vi "PicoScope5000aSettings.vi"(0 "error in":errorcluster, 1 "Channel A Settings":T2={"Enabled"=FALSE, "Coupling"=1, "Range"=6, "Analogue Offset"=0.0, "Bandwidth Limit"=0} {"Bandwidth Limit" items=["Full", "20MHz"]; "Range" items=["10 mV", "20 mV", "50 mV", "100 mV", "200 mV", "500 mV", "1 V", "2 V", "5 V", "10 V", "20 V"]; "Coupling" items=["AC", "DC"]}, 2 "Port 0 Settings":cluster{"Enabled":bool, "Logic Level":i16}={"Enabled"=FALSE, "Logic Level"=9830} {"Logic Level" items=["1.5V TTL"=9830, "2.5V CMOS"=16383]}, 3 "Channel B Settings":T2={"Enabled"=FALSE, "Coupling"=1, "Range"=6, "Analogue Offset"=0.0, "Bandwidth Limit"=0} {"Bandwidth Limit" items=["Full", "20MHz"]; "Range" items=["10 mV", "20 mV", "50 mV", "100 mV", "200 mV", "500 mV", "1 V", "2 V", "5 V", "10 V", "20 V"]; "Coupling" items=["AC", "DC"]}, 5 "handle in":i16, 9 "Device Info":T1, 11 "Trigger Settings":T3={"Trigger Enabled"=FALSE, "Trigger Source"=enum."Channel A", "Trigger Threshold (volts)"=0.0, "Trigger Direction"=2, "Trigger Delay (samples)"=0, "Auto Trigger Time (ms)"=1000} {"Trigger Direction" items=["Rising"=2, "Falling"=3]}, 12 "Channel C Settings":T2={"Enabled"=FALSE, "Coupling"=1, "Range"=6, "Analogue Offset"=0.0, "Bandwidth Limit"=0} {"Bandwidth Limit" items=["Full", "20MHz"]; "Range" items=["10 mV", "20 mV", "50 mV", "100 mV", "200 mV", "500 mV", "1 V", "2 V", "5 V", "10 V", "20 V"]; "Coupling" items=["AC", "DC"]}, 13 "Port 1 Settings":cluster{"Enabled":bool, "Logic Level":i16}={"Enabled"=FALSE, "Logic Level"=9830} {"Logic Level" items=["1.5V TTL"=9830, "2.5V CMOS"=16383]}, 14 "Channel D Settings":T2={"Enabled"=FALSE, "Coupling"=1, "Range"=6, "Analogue Offset"=0.0, "Bandwidth Limit"=0} {"Bandwidth Limit" items=["Full", "20MHz"]; "Range" items=["10 mV", "20 mV", "50 mV", "100 mV", "200 mV", "500 mV", "1 V", "2 V", "5 V", "10 V", "20 V"]; "Coupling" items=["AC", "DC"]}, 15 "Max ADC value":i16) -> (4 "error out":errorcluster, 6 "handle out":i16, 8 "enabled array":i16[](array[numeric]))   [LabVIEW 2020]
doc: "This VI is used to set up the oscilloscope. The inputs are clusters for setting channel and simple trigger settings. Advanced triggers can be set up using PicoScope3000aAdvancedTriggerSettings.vi"
uses:
  ps5000a.dll
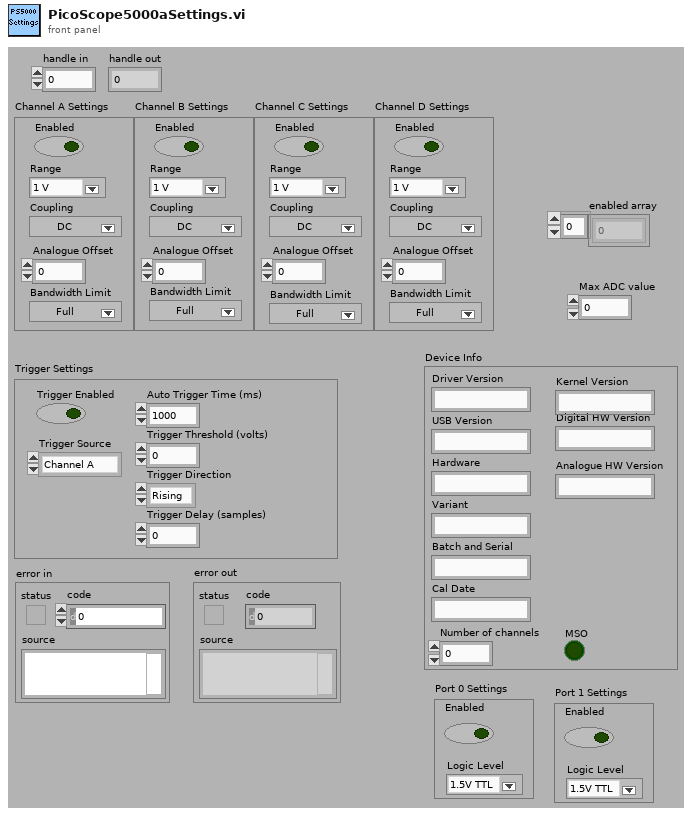
[diagram p1: front panel]
types:
  T1 = cluster{"Driver Version":string, "USB Version":string, "Hardware":string, "Variant":string, "Batch and Serial":string, "Cal Date":string, "Kernel Version":string, "Digital HW Version":string, "Analogue HW Version":string, "MSO":bool, "Number of channels":i16}
  T2 = cluster{"Enabled":bool, "Coupling":i16, "Range":u16, "Analogue Offset":sgl, "Bandwidth Limit":u32}
  T3 = cluster{"Trigger Enabled":bool, "Trigger Source":enum16{"Channel A", "Channel B", "Channel C", "Channel D", "Ext."}, "Trigger Threshold (volts)":dbl, "Trigger Direction":u16, "Trigger Delay (samples)":u32, "Auto Trigger Time (ms)":i16}
  T4 = enum16{"Channel A", "Channel B", "Channel C", "Channel D", "Ext."}
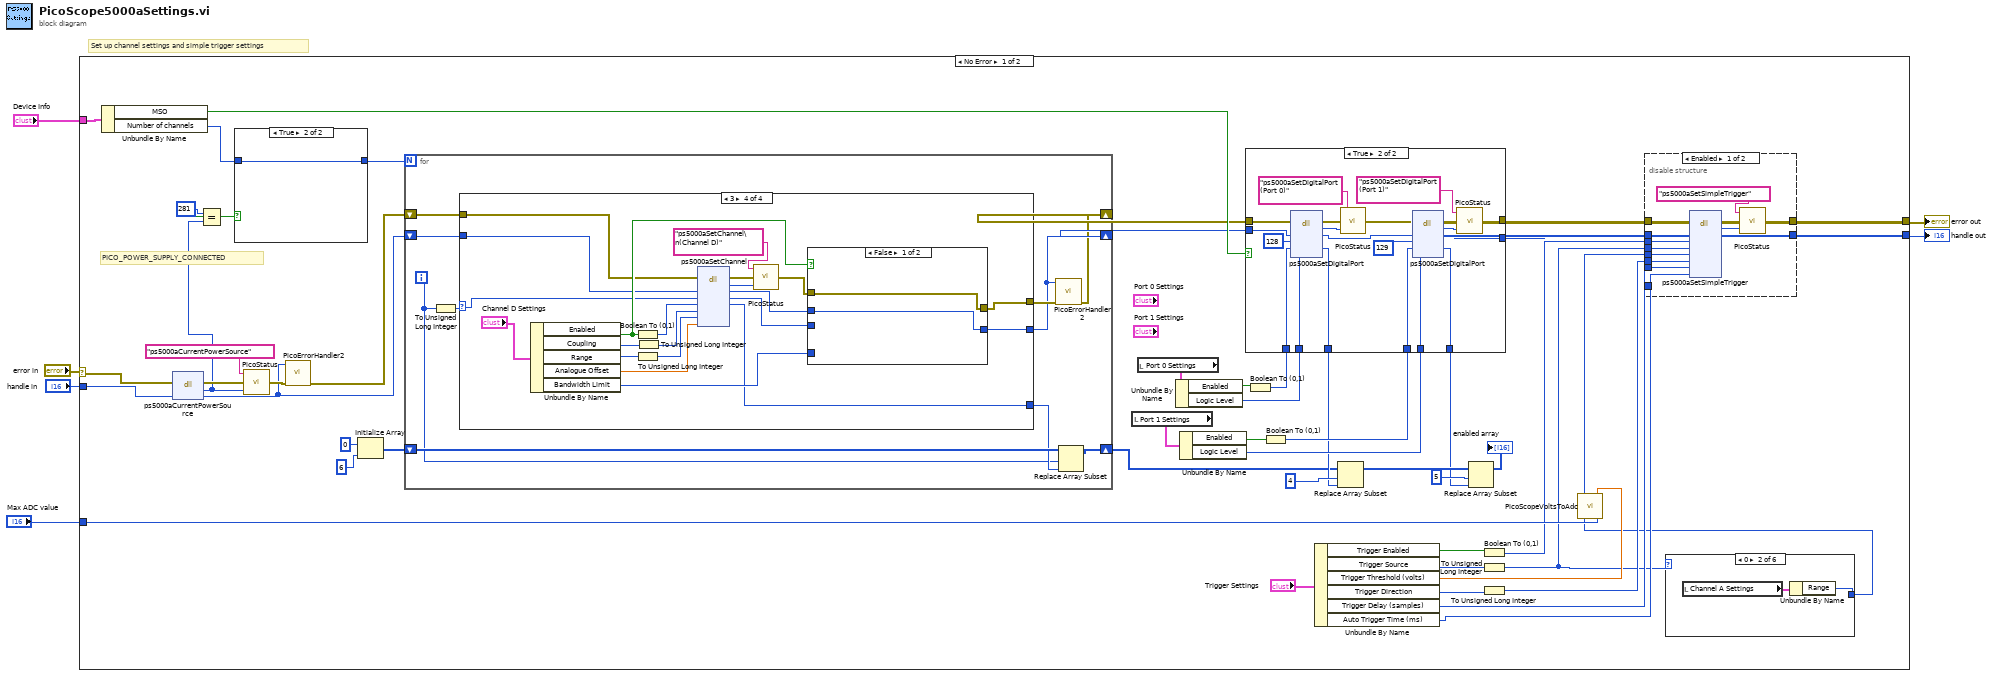
[diagram p0: block diagram]
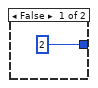
[diagram p3: hidden frame]
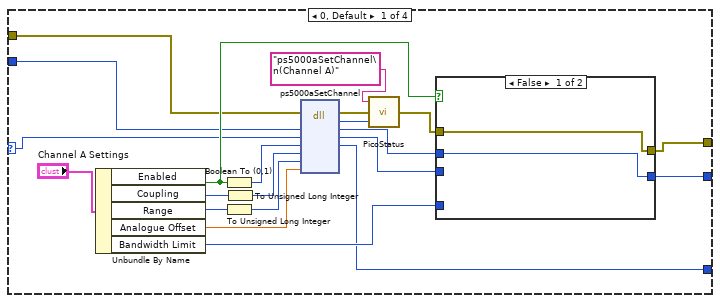
[diagram p4: hidden frame]
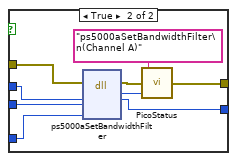
[diagram p5: hidden frame]
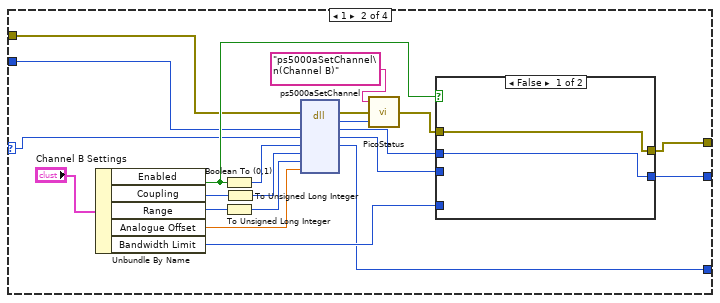
[diagram p6: hidden frame]
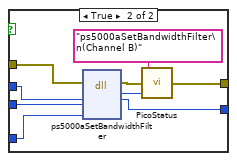
[diagram p7: hidden frame]
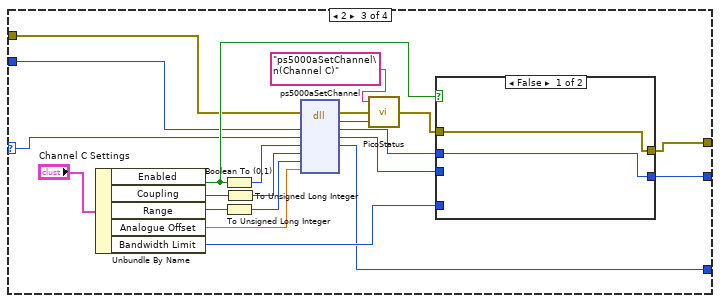
[diagram p8: hidden frame]
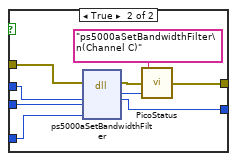
[diagram p9: hidden frame]
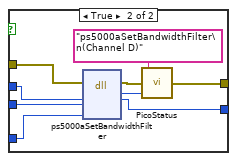
[diagram p10: hidden frame]
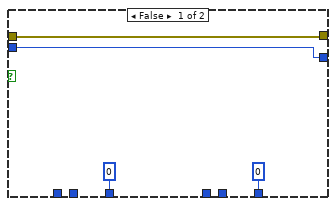
[diagram p11: hidden frame]
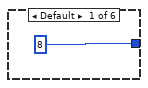
[diagram p12: hidden frame]
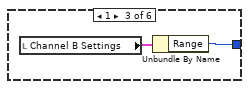
[diagram p13: hidden frame]
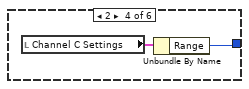
[diagram p14: hidden frame]
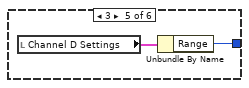
[diagram p15: hidden frame]
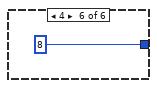
[diagram p16: hidden frame]
diagram:
  # "Set up channel settings and simple trigger settings"
  n1 = case shown="No Error" "error in" {
    selector: "error in" -> [w16 w248]
    tunnel: "handle in" -> [w15 w247]
    tunnel: [w51 w247] -> w4
    tunnel: [w41 w248] -> w3
    tunnel: "Device Info" -> [w46 _]
    tunnel: "Max ADC value" -> [w43 _]
    frame No Error {
      # "PICO_POWER_SUPPLY_CONNECTED"
      n2 = Unbundle By Name(w46) -> ("MSO"=w23:bool, "Number of channels"=w10:i16)
      n3 = dll-call lib="ps5000a.dll" fn="ps5000aCurrentPowerSource"(error in=w16, "handle"=w15) -> (error out=w49:errorcluster, "PICO_STATUS"=w47:u32, "handle"=w13:i16)  [unwired: 2 in, 1 out]
      n4 = Equal?(x=u32 281, y=w47) -> (x = y?=w11:bool)
      n5 = case shown="True" w11 {
        tunnel: [i16 2 ("Number of channels") w74] -> w8
        tunnel: w10 -> [_ w74]
        frame False {
        }
        frame True {
        }
      }
      n6 = call "PicoStatus.vi"("PICO STATUS"=w47, "error in"=w49, "source"="ps5000aCurrentPowerSource") -> ("error out"=w14:errorcluster)
      n7 = call "PicoErrorHandler2.vi"("error in (no error)"=w14, "handle In"=w13) -> ("error out"=w12:errorcluster)  [unwired: 9 in]
      n8 = Initialize Array(i16 0 ("element"), 6 ("dimension size")) -> (w20:i16[])
      n9 = for {
        N: w8 -> [_]
        shift-right: [w82] -> w19
        shift-left: w20 -> [w84]
        shift-right: [w79] -> w18
        shift-left: w12 -> [w81]
        shift-right: [w77] -> w17
        shift-left: w13 -> [w80]
        i -> [w75]
        n10 = To Unsigned Long Integer(number=w75) -> (unsigned 32bit integer=w76:u32)
        n11 = case shown="3" w76 {
          selector: w76 -> [w85 w117 w149 w181]
          tunnel: [w90 w123 w155 w187] -> w83
          tunnel: w81 -> [w89 w121 w153 w185]
          tunnel: w80 -> [w88 w120 w152 w184]
          tunnel: [w87 w119 w151 w183] -> w78
          tunnel: [w86 w118 w150 w182] -> w77
          frame 0, Default {
            n12 = Unbundle By Name("Channel A Settings") -> ("Enabled"=w94:bool, "Coupling"=w104:i16, "Range"=w105:u16, "Analogue Offset"=w102:sgl, "Bandwidth Limit"=w95:u32)
            n13 = Boolean To (0,1)(Boolean=w94) -> (0, 1=w97:i16)
            n14 = To Unsigned Long Integer(number=w105) -> (unsigned 32bit integer=w101:u32)
            n15 = To Unsigned Long Integer(number=w104) -> (unsigned 32bit integer=w103:u32)
            n16 = dll-call lib="ps5000a.dll" fn="ps5000aSetChannel" ("ps3000.dll:_ps3000_open_unit@0")(error in=w89, "handle"=w88, "channel"=w85, "enabled"=w97, "dc"=w103, "range"=w101, "analogueOffset"=w102) -> (error out=w100:errorcluster, "PICO_STATUS"=w99:u32, "handle"=w92:i16, "channel"=w91:u32, "enabled"=w90:i16)  [unwired: 5 in, 1 out]
            n17 = call "PicoStatus.vi"("PICO STATUS"=w99, "error in"=w100, "source"="ps5000aSetChannel\n(Channel A)") -> ("error out"=w93:errorcluster)
            n18 = case shown="False" w94 {
              tunnel: w93 -> [w107 w113]
              tunnel: [w107 w112] -> w87
              tunnel: [w106 w111] -> w86
              tunnel: w91 -> [_ w110]
              tunnel: w92 -> [w106 w109]
              tunnel: w95 -> [_ w108]
              frame False {
              }
              frame True {
                n19 = dll-call lib="ps5000a.dll" fn="ps5000aSetBandwidthFilter" ("ps3000.dll:_ps3000_open_unit@0")(error in=w113, "handle"=w109, "channel"=w110, "Bandwidth Limit"=w108) -> (error out=w115:errorcluster, "PICO_STATUS"=w114:u32, "handle"=w111:i16)  [unwired: 4 in, 1 out]
                n20 = call "PicoStatus.vi"("PICO STATUS"=w114, "error in"=w115, "source"="ps5000aSetBandwidthFilter\n(Channel A)") -> ("error out"=w112:errorcluster)
              }
            }
          }
          frame 1 {
            n21 = Unbundle By Name("Channel B Settings") -> ("Enabled"=w127:bool, "Coupling"=w136:i16, "Range"=w137:u16, "Analogue Offset"=w134:sgl, "Bandwidth Limit"=w128:u32)
            n22 = Boolean To (0,1)(Boolean=w127) -> (0, 1=w130:i16)
            n23 = To Unsigned Long Integer(number=w137) -> (unsigned 32bit integer=w133:u32)
            n24 = To Unsigned Long Integer(number=w136) -> (unsigned 32bit integer=w135:u32)
            n25 = dll-call lib="ps5000a.dll" fn="ps5000aSetChannel" ("ps3000.dll:_ps3000_open_unit@0")(error in=w121, "handle"=w120, "channel"=w117, "enabled"=w130, "dc"=w135, "range"=w133, "analogueOffset"=w134) -> (error out=w132:errorcluster, "PICO_STATUS"=w131:u32, "handle"=w125:i16, "channel"=w124:u32, "enabled"=w123:i16)  [unwired: 5 in, 1 out]
            n26 = call "PicoStatus.vi"("PICO STATUS"=w131, "error in"=w132, "source"="ps5000aSetChannel\n(Channel B)") -> ("error out"=w126:errorcluster)
            n27 = case shown="False" w127 {
              tunnel: w126 -> [w139 w145]
              tunnel: [w139 w144] -> w119
              tunnel: [w138 w143] -> w118
              tunnel: w124 -> [_ w142]
              tunnel: w125 -> [w138 w141]
              tunnel: w128 -> [_ w140]
              frame False {
              }
              frame True {
                n28 = dll-call lib="ps5000a.dll" fn="ps5000aSetBandwidthFilter" ("ps3000.dll:_ps3000_open_unit@0")(error in=w145, "handle"=w141, "channel"=w142, "Bandwidth Limit"=w140) -> (error out=w147:errorcluster, "PICO_STATUS"=w146:u32, "handle"=w143:i16)  [unwired: 4 in, 1 out]
                n29 = call "PicoStatus.vi"("PICO STATUS"=w146, "error in"=w147, "source"="ps5000aSetBandwidthFilter\n(Channel B)") -> ("error out"=w144:errorcluster)
              }
            }
          }
          frame 2 {
            n30 = Unbundle By Name("Channel C Settings") -> ("Enabled"=w159:bool, "Coupling"=w168:i16, "Range"=w169:u16, "Analogue Offset"=w166:sgl, "Bandwidth Limit"=w160:u32)
            n31 = Boolean To (0,1)(Boolean=w159) -> (0, 1=w162:i16)
            n32 = To Unsigned Long Integer(number=w169) -> (unsigned 32bit integer=w165:u32)
            n33 = To Unsigned Long Integer(number=w168) -> (unsigned 32bit integer=w167:u32)
            n34 = dll-call lib="ps5000a.dll" fn="ps5000aSetChannel" ("ps3000.dll:_ps3000_open_unit@0")(error in=w153, "handle"=w152, "channel"=w149, "enabled"=w162, "dc"=w167, "range"=w165, "analogueOffset"=w166) -> (error out=w164:errorcluster, "PICO_STATUS"=w163:u32, "handle"=w157:i16, "channel"=w156:u32, "enabled"=w155:i16)  [unwired: 5 in, 1 out]
            n35 = call "PicoStatus.vi"("PICO STATUS"=w163, "error in"=w164, "source"="ps5000aSetChannel\n(Channel C)") -> ("error out"=w158:errorcluster)
            n36 = case shown="False" w159 {
              tunnel: w158 -> [w171 w177]
              tunnel: [w171 w176] -> w151
              tunnel: [w170 w175] -> w150
              tunnel: w156 -> [_ w174]
              tunnel: w157 -> [w170 w173]
              tunnel: w160 -> [_ w172]
              frame False {
              }
              frame True {
                n37 = dll-call lib="ps5000a.dll" fn="ps5000aSetBandwidthFilter" ("ps3000.dll:_ps3000_open_unit@0")(error in=w177, "handle"=w173, "channel"=w174, "Bandwidth Limit"=w172) -> (error out=w179:errorcluster, "PICO_STATUS"=w178:u32, "handle"=w175:i16)  [unwired: 4 in, 1 out]
                n38 = call "PicoStatus.vi"("PICO STATUS"=w178, "error in"=w179, "source"="ps5000aSetBandwidthFilter\n(Channel C)") -> ("error out"=w176:errorcluster)
              }
            }
          }
          frame 3 {
            n39 = Unbundle By Name("Channel D Settings") -> ("Enabled"=w191:bool, "Coupling"=w200:i16, "Range"=w201:u16, "Analogue Offset"=w198:sgl, "Bandwidth Limit"=w192:u32)
            n40 = Boolean To (0,1)(Boolean=w191) -> (0, 1=w194:i16)
            n41 = To Unsigned Long Integer(number=w201) -> (unsigned 32bit integer=w197:u32)
            n42 = To Unsigned Long Integer(number=w200) -> (unsigned 32bit integer=w199:u32)
            n43 = dll-call lib="ps5000a.dll" fn="ps5000aSetChannel" ("ps3000.dll:_ps3000_open_unit@0")(error in=w185, "handle"=w184, "channel"=w181, "enabled"=w194, "dc"=w199, "range"=w197, "analogueOffset"=w198) -> (error out=w196:errorcluster, "PICO_STATUS"=w195:u32, "handle"=w189:i16, "channel"=w188:u32, "enabled"=w187:i16)  [unwired: 5 in, 1 out]
            n44 = call "PicoStatus.vi"("PICO STATUS"=w195, "error in"=w196, "source"="ps5000aSetChannel\n(Channel D)") -> ("error out"=w190:errorcluster)
            n45 = case shown="False" w191 {
              tunnel: w190 -> [w203 w209]
              tunnel: [w203 w208] -> w183
              tunnel: [w202 w207] -> w182
              tunnel: w188 -> [_ w206]
              tunnel: w189 -> [w202 w205]
              tunnel: w192 -> [_ w204]
              frame False {
              }
              frame True {
                n46 = dll-call lib="ps5000a.dll" fn="ps5000aSetBandwidthFilter" ("ps3000.dll:_ps3000_open_unit@0")(error in=w209, "handle"=w205, "channel"=w206, "Bandwidth Limit"=w204) -> (error out=w211:errorcluster, "PICO_STATUS"=w210:u32, "handle"=w207:i16)  [unwired: 4 in, 1 out]
                n47 = call "PicoStatus.vi"("PICO STATUS"=w210, "error in"=w211, "source"="ps5000aSetBandwidthFilter\n(Channel D)") -> ("error out"=w208:errorcluster)
              }
            }
          }
        }
        n48 = call "PicoErrorHandler2.vi"("error in (no error)"=w78, "handle In"=w77) -> ("error out"=w79:errorcluster)  [unwired: 9 in]
        n49 = Replace Array Subset(array=w84, new element=w83, index=w75) -> (w82:i16[])
      }
      n50 = local read "Port 1 Settings"() -> (w39:cluster{"Enabled":bool, "Logic Level":i16})
      n51 = local read "Port 0 Settings"() -> (w40:cluster{"Enabled":bool, "Logic Level":i16})
      n52 = Unbundle By Name(w40) -> ("Enabled"=w38:bool, "Logic Level"=w36:i16)
      n53 = Unbundle By Name(w39) -> ("Enabled"=w35:bool, "Logic Level"=w33:i16)
      n54 = Boolean To (0,1)(Boolean=w38) -> (0, 1=w37:i16)
      n55 = Boolean To (0,1)(Boolean=w35) -> (0, 1=w34:i16)
      n56 = case shown="True" w23 {
        tunnel: [w216 w228] -> w32
        tunnel: w37 -> [_ w225]
        tunnel: w36 -> [_ w224]
        tunnel: w34 -> [_ w223]
        tunnel: w33 -> [_ w222]
        tunnel: w18 -> [w216 w221]
        tunnel: w17 -> [w215 w220]
        tunnel: [w215 w219] -> w31
        tunnel: [i16 0 ("enabled") w218] -> w26
        tunnel: [i16 0 ("enabled") w217] -> w25
        frame False {
        }
        frame True {
          n57 = dll-call lib="PS5000a.dll" fn="ps5000aSetDigitalPort"(error in=w221, "handle"=w220, "port"=u32 128, "enabled"=w225, "logicLevel"=w224) -> (error out=w236:errorcluster, "PICO_STATUS"=w233:u32, "handle"=w229:i16, "enabled"=w218:i16)  [unwired: 4 in, 1 out]
          n58 = call "PicoStatus.vi"("PICO STATUS"=w233, "error in"=w236, "source"="ps5000aSetDigitalPort (Port 0)") -> ("error out"=w230:errorcluster)
          n59 = dll-call lib="PS5000a.dll" fn="ps5000aSetDigitalPort"(error in=w230, "handle"=w229, "port"=u32 129, "enabled"=w223, "logicLevel"=w222) -> (error out=w232:errorcluster, "PICO_STATUS"=w231:u32, "handle"=w219:i16, "enabled"=w217:i16)  [unwired: 4 in, 1 out]
          n60 = call "PicoStatus.vi"("PICO STATUS"=w231, "error in"=w232, "source"="ps5000aSetDigitalPort (Port 1)") -> ("error out"=w228:errorcluster)
        }
      }
      n61 = Unbundle By Name("Trigger Settings") -> ("Trigger Enabled"=w52:bool, "Trigger Source"=w53:T4, "Trigger Threshold (volts)"=w44:dbl, "Trigger Direction"=w55:u16, "Trigger Delay (samples)"=w54:u32, "Auto Trigger Time (ms)"=w42:i16)
      n62 = Replace Array Subset(array=w19, new element=w26, index=4) -> (w27:i16[])
      n63 = Replace Array Subset(array=w27, new element=w25, index=5) -> (→"enabled array":i16[])
      n64 = Boolean To (0,1)(Boolean=w52) -> (0, 1=w30:i16)
      n65 = To Unsigned Long Integer(number=w53) -> (unsigned 32bit integer=w7:u32)
      n66 = To Unsigned Long Integer(number=w55) -> (unsigned 32bit integer=w57:u32)
      n67 = case shown="0" w7 {
        tunnel: [u16 8 ("Range") w238 w240 w242 w244 u16 8 ("Range")] -> w9
        frame Default {
        }
        frame 0 {
          n68 = local read "Channel A Settings"() -> (w239:T2)
          n69 = Unbundle By Name(w239) -> ("Range"=w238:u16)
        }
        frame 1 {
          n70 = local read "Channel B Settings"() -> (w241:T2)
          n71 = Unbundle By Name(w241) -> ("Range"=w240:u16)
        }
        frame 2 {
          n72 = local read "Channel C Settings"() -> (w243:T2)
          n73 = Unbundle By Name(w243) -> ("Range"=w242:u16)
        }
        frame 3 {
          n74 = local read "Channel D Settings"() -> (w245:T2)
          n75 = Unbundle By Name(w245) -> ("Range"=w244:u16)
        }
        frame 4 {
        }
      }
      n76 = call "PicoScopeVoltsToAdc.vi"("Max_adc"=w43, "Volts"=w44, "Range Index"=w9) -> ("ADC count"=w45:i16)
      n77 = disable-structure shown="Enabled" {
        disable-tunnel: w57 -> [w70 _]
        disable-tunnel: w54 -> [w69 _]
        disable-tunnel: [w65 w72] -> w51
        disable-tunnel: w45 -> [w64 _]
        disable-tunnel: w42 -> [w63 _]
        disable-tunnel: [w62 w71] -> w41
        disable-tunnel: w32 -> [w61 w71]
        disable-tunnel: w31 -> [w60 w72]
        disable-tunnel: w30 -> [w59 _]
        disable-tunnel: w7 -> [w58 _]
        frame Enabled {
          n78 = dll-call lib="ps5000a.dll" fn="ps5000aSetSimpleTrigger" ("ps3000.dll:_ps3000_open_unit@0")(error in=w61, "handle"=w60, "enable"=w59, "source"=w58, "threshold"=w64, "direction"=w70, "delay"=w69, "autoTrigger_ms"=w63) -> (error out=w67:errorcluster, "PICO_STATUS"=w68:u32, "handle"=w65:i16)  [unwired: 8 in, 1 out]
          n79 = call "PicoStatus.vi"("PICO STATUS"=w68, "error in"=w67, "source"="ps5000aSetSimpleTrigger") -> ("error out"=w62:errorcluster)
        }
        frame Disabled {
        }
      }
    }
    frame Error {
    }
  }
  "handle out" <- w4
  "error out" <- w3
